vi "Cam Grab (SubVI).vi"(8 "error in (no error)":errorcluster, 10 "Image in":T1, 11 "Cam Ref":T2) -> (0 "error out":errorcluster, 1 "Image Pixels (U32)":u32[][](array[numeric]), 2 "Image out":T1, 3 "Session out":T2)   [LabVIEW 2013]
uses:
  <vilib>/vision/Image Controls.llb/IMAQ Image.ctl
  <vilib>/userdefined/High Color/IMAQdx.ctl
  <vilib>/vision/driver/IMAQdx.llb/IMAQdx Buffer Number Mode.ctl
  <vilib>/vision/driver/NI_Vision_Acquisition_Software.lvlib
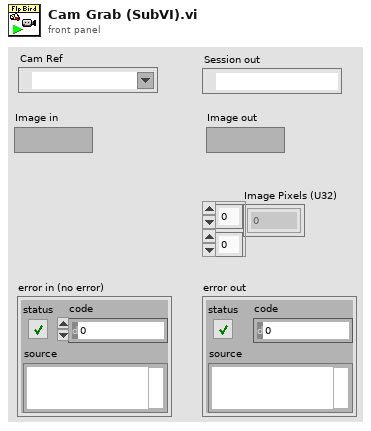
[diagram p1: front panel]
types:
  T1 = typedef "IMAQ Image.ctl" = refnum<image>
  T2 = typedef "IMAQdx.ctl" = refnum<k21>
  T3 = typedef "NI_Vision_Acquisition_Software.lvlib/IMAQdx Buffer Number Mode.ctl" = enum32{"Next", "Last", "Buffer Number"}
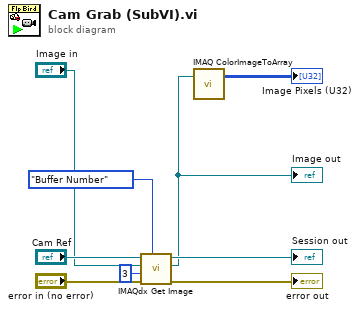
[diagram p0: block diagram]
diagram:
  n1 = call <vilib>:"IMAQdx Get Image.vi"("Buffer Number Mode (Next)"=IMAQdx_Buffer_Number_Mode."Buffer Number", "error in"="error in (no error)", "Buffer Number In"=u32 3, "Image In"="Image in", "Session In"="Cam Ref") -> ("error out"=→"error out":errorcluster, "Image Out"=w1:T1, "Session Out"=→"Session out":T2)  [unwired: 3 in, 1 out]
  "Image out" <- w1
  n2 = call "IMAQ ColorImageToArray"("Image"=w1) -> ("Image Pixels (U32)"=→"Image Pixels (U32)":u32[][])  [unwired: 3 in, 2 out]
